vi "Read Hex Path.vi"(8 "error in":errorcluster, 11 "MPLab in":refnum<class "MPLab.lvclass">) -> (0 "error out":errorcluster, 3 "MPLab out":refnum<class "MPLab.lvclass">)   [LabVIEW 2018, in "MPLab.lvlib" / "MPLab.lvclass"]
uses:
  MPLab.lvclass
  MPLab.lvclass/MPLab.ctl
  builds/Configuration.lvlibp/Configuration.lvclass
  builds/Flash Utility.lvlibp/Flash Utility.lvclass
  C:/Users/Ron.Dexter.LUMINARTECH/Desktop/builds/Flash Utility.lvlibp/Flash Utility.lvclass
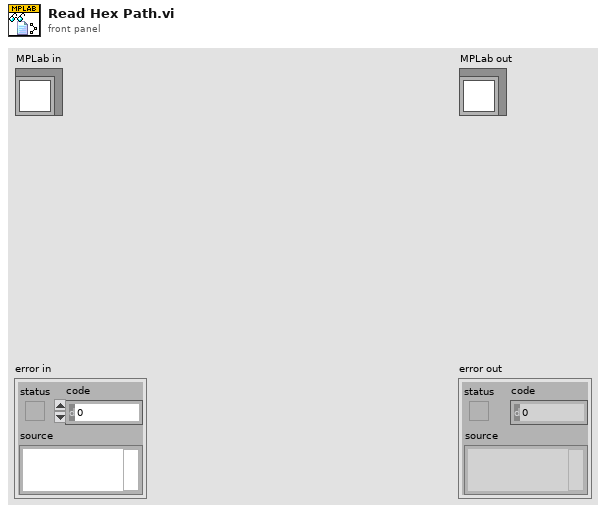
[diagram p1: front panel]
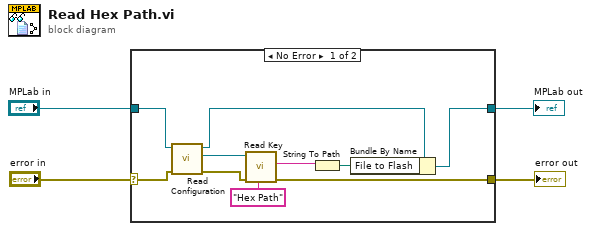
[diagram p0: block diagram]
diagram:
  n1 = case shown="No Error" "error in" {
    selector: "error in" -> [w10 w16]
    tunnel: [w9 w16] -> w3
    tunnel: [w5 w15] -> w1
    tunnel: "MPLab in" -> [w6 w15]
    frame No Error {
      n2 = call "Read Configuration.vi"("error in (no error)"=w10, "Flash Utility in"=w6) -> ("error out"=w11:errorcluster, "Configuration"=w14:refnum<class "Configuration.lvclass">, "Flash Utility out"=w7:refnum<class "MPLab.lvclass">)  [unwired: 7 in]
      n3 = call "Read Key.vi"("Key:"="Hex Path", "error in"=w11, "Configuration in"=w14) -> ("error out"=w9:errorcluster, "Value"=w13:string)  [unwired: 6 in, 1 out]
      n4 = String To Path(string=w13) -> (path=w8:path)
      n5 = Bundle By Name(cluster=w7, "File to Flash"=w8) -> (w5:refnum<class "MPLab.lvclass">)
    }
    frame Error {
    }
  }
  "error out" <- w3
  "MPLab out" <- w1
